vi "Handle Command.vi"(8 "error in (no error)":errorcluster, 9 "Data":variant, 10 "Command":string, 11 "instrument.Cryostation in":refnum<class "instrument.Cryostation.lvclass">) -> (0 "error out":errorcluster, 1 "Processed Data":variant, 2 "Command":string, 3 "instrument.Cryostation out":refnum<class "instrument.Cryostation.lvclass">)   [LabVIEW 2016, in "instrument.Cryostation.lvclass"]
uses:
  instrument.Cryostation.lvclass
  instrument.Cryostation.lvclass/instrument.Cryostation.ctl
  <userlib>/LevyLab/Levylab Instruments/Instrument Types/Cryostat/Instrument.Cryostat.lvclass
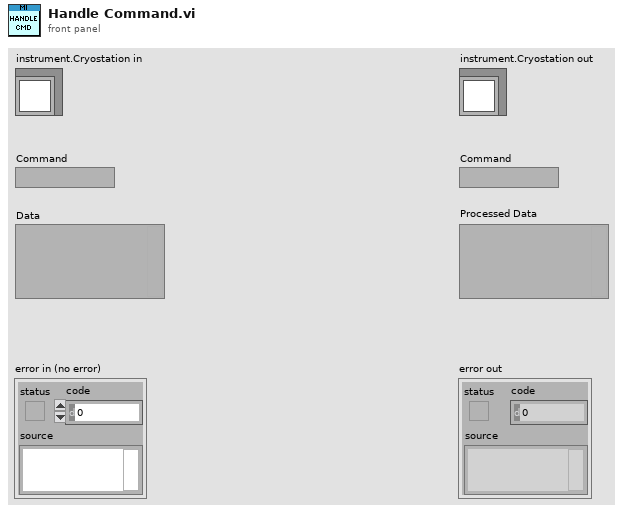
[diagram p1: front panel]
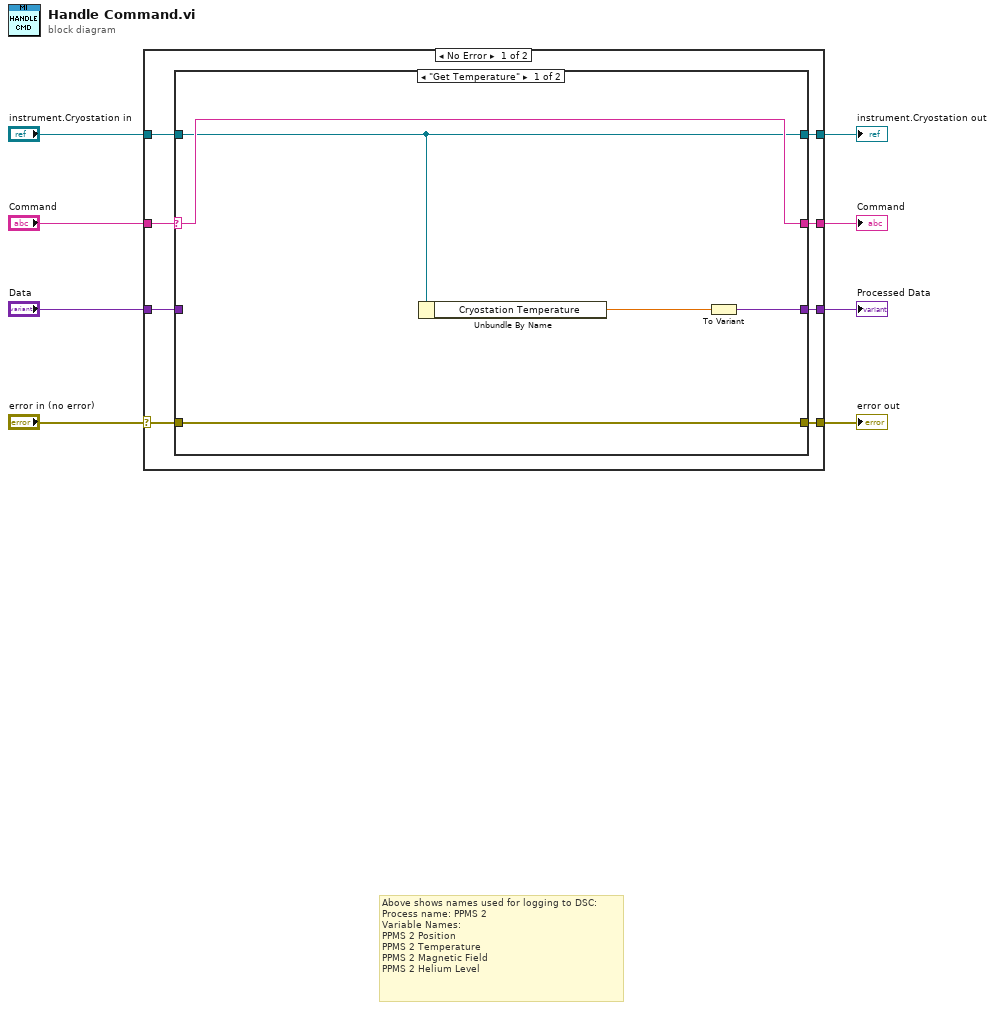
[diagram p0: block diagram]
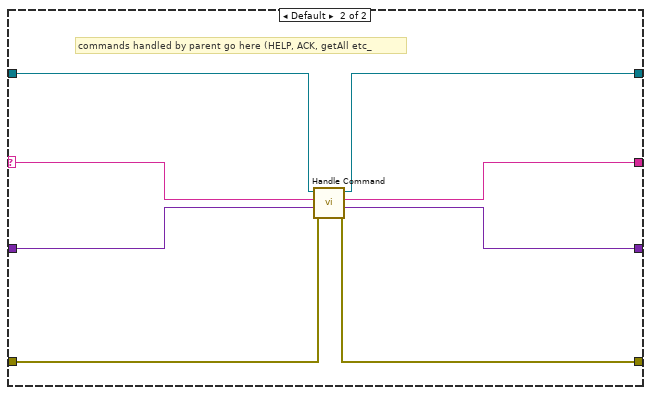
[diagram p2: hidden frame]
diagram:
  # "Above shows names used for logging to DSC:\nProcess name: PPMS 2\nVariable Names:\nPPMS 2 Position\nPPMS 2 Temperature\nPPMS 2 Magnetic Field\nPPMS 2 Helium Level"
  n1 = case shown="No Error" "error in (no error)" {
    selector: "error in (no error)" -> [w11 w30]
    tunnel: [w10 w30] -> w6
    tunnel: [w16 _] -> w4
    tunnel: [w15 _] -> w5
    tunnel: [w14 w31] -> w7
    tunnel: "Data" -> [w13 _]
    tunnel: "Command" -> [w9 _]
    tunnel: "instrument.Cryostation in" -> [w12 w31]
    frame No Error {
      n2 = case shown="\"Get Temperature\"" w9 {
        selector: w9 -> [w20 w22]
        tunnel: [w21 w29] -> w16
        tunnel: [w20 w28] -> w15
        tunnel: [w17 w27] -> w14
        tunnel: w13 -> [_ w26]
        tunnel: w12 -> [w17 w25]
        tunnel: w11 -> [w19 w24]
        tunnel: [w19 w23] -> w10
        frame "Get Temperature" {
          n3 = Unbundle By Name(w17) -> ("Cryostation Temperature"=w18:dbl)
          n4 = To Variant(anything=w18) -> (Variant=w21:variant)
        }
        frame Default {
          # "commands handled by parent go here (HELP, ACK, getAll etc_"
          n5 = call-parent "Handle Command.vi"("error in (no error)"=w24, "Data"=w26, "Command"=w22, "Instrument in"=w25) -> ("error out"=w23:errorcluster, "Processed Data"=w29:variant, "Command"=w28:string, "Instrument out"=w27:refnum<class "instrument.Cryostation.lvclass">)  [unwired: 4 in]
        }
      }
    }
    frame Error {
    }
  }
  "error out" <- w6
  "instrument.Cryostation out" <- w7
  "Processed Data" <- w4
  "Command" <- w5
